vi "灯值调整对话框.vi"() -> ()   [LabVIEW 2016, in "斯坦道氨氮.lvlib"]
uses:
  <vilib>/Plasmionique/MB Master/MB_Master/MB_Master.lvclass
panel:
  out "工作状态:":string
  in  "纯水填充":bool
  out "660 阻值":u16 caption="660 阻值："
  out "520 阻值":u16 caption="520 阻值："
  out "365 阻值":u16 caption="365 阻值："
  in  "停止":bool
  in  "校准":bool
  out "校准状态":u16(ring) caption="调灯状态：" items=["空闲", "校准中"]
  out "当前阻值":u16 caption="当前阻值："
  out "当前光强":u16 caption="当前光强："
  in  "目标光强":u16=3300 caption="目标光强："
  in  "灯类型":enum32{"365", "520", "660"}(radio)=enum."660" caption="灯类型："
  # "365：营养盐\n520：营养盐、氨氮总磷-氨氮光源\n660：总磷、氨氮"
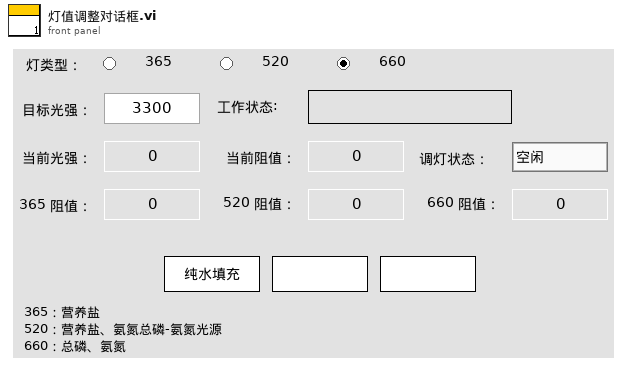
[diagram p1: front panel]
types:
  T1 = cluster{"360 阻值":u16, "520 阻值":u16, "660 阻值":u16}
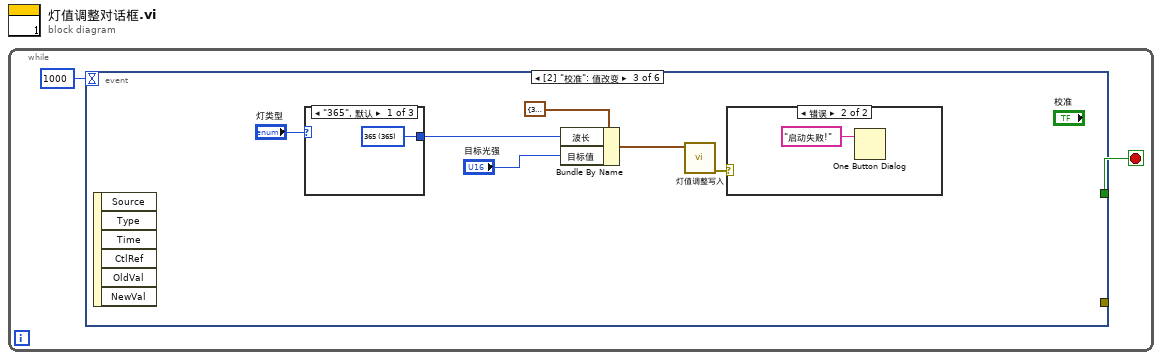
[diagram p0: block diagram]
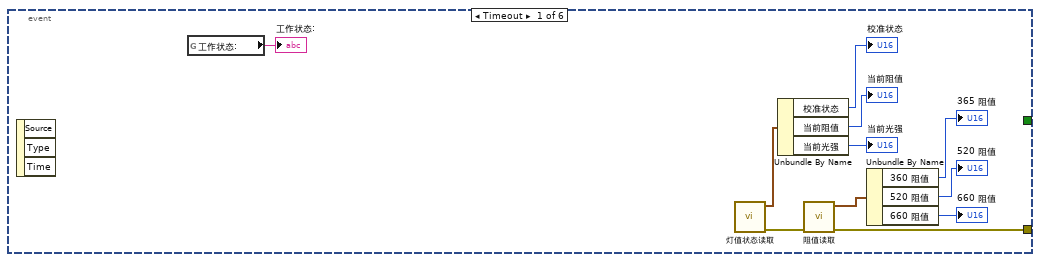
[diagram p2: hidden frame]
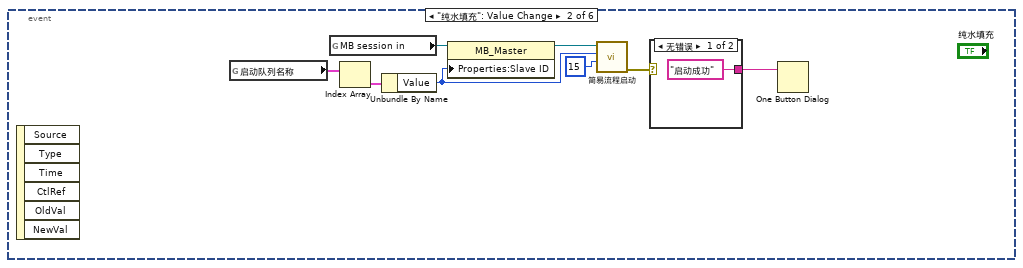
[diagram p3: hidden frame]
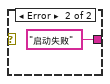
[diagram p4: hidden frame]
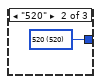
[diagram p6: hidden frame]
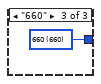
[diagram p7: hidden frame]
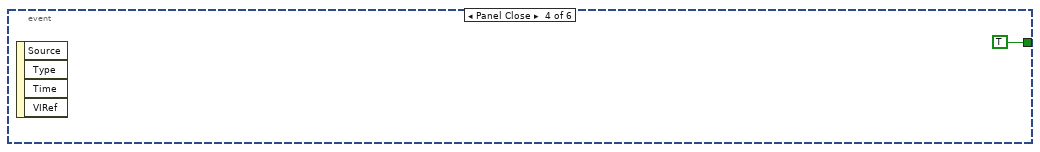
[diagram p8: hidden frame]
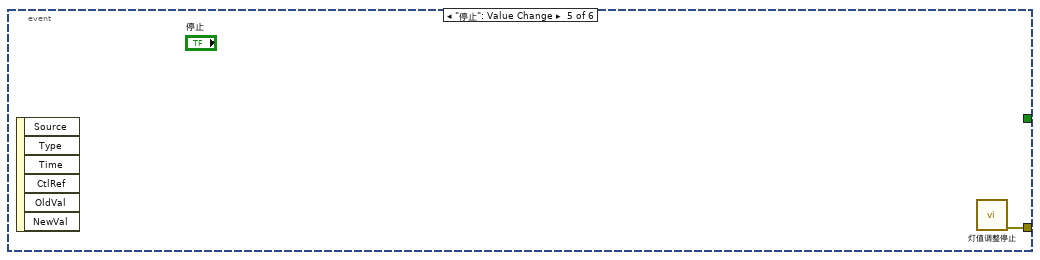
[diagram p9: hidden frame]
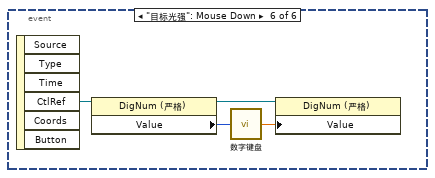
[diagram p10: hidden frame]
diagram:
  n1 = while {
    stop <- w2 stop-if-true
    n2 = event shown="[2] \"校准\": 值改变" {
      selector: _ -> [_ _ _ _ _ _]
      dyn-events: _ -> [_ _ _ _ _ _]
      timeout: 1000 -> [_ _ _ _ _ _]
      tunnel: [_ _ _ TRUE _ _] -> w2
      tunnel: [w4 _ _ _ w35 _] -> _
      event Timeout {
        n3 = event-data() -> ()  [unwired: 1 in, 3 out]
        n4 = global read "VAR总磷总氮全局变量.vi" "工作状态:"() -> (→"工作状态:":string)
        n5 = call "灯值状态读取.vi"() -> ("error out"=w13:errorcluster, "状态值"=w12:cluster{"校准状态":u16, "当前阻值":u16, "当前光强":u16})  [unwired: 10 in]
        n6 = Unbundle By Name(w12) -> ("校准状态"=→"校准状态":u16, "当前阻值"=→"当前阻值":u16, "当前光强"=→"当前光强":u16)
        n7 = call "阻值读取.vi"("error in (no error)"=w13) -> ("error out"=w4:errorcluster, "状态值"=w8:T1)  [unwired: 9 in]
        n8 = Unbundle By Name(w8) -> ("360 阻值"=→"365 阻值":u16, "520 阻值"=→"520 阻值":u16, "660 阻值"=→"660 阻值":u16)
      }
      event "纯水填充": Value Change {
        n9 = event-data() -> ()  [unwired: 1 in, 6 out]
        n10 = global read "总磷总氮断电保存全局变量.vi" "启动队列名称"() -> (w16:cluster{"String":string, "Value":u16}[])
        n11 = global read "VAR总磷总氮全局变量.vi" "MB session in"() -> (w19:refnum<class "MB_Master.lvclass">)
        n12 = Index Array(array=w16) -> (element=w15:cluster{"String":string, "Value":u16})  [unwired: 1 in]
        n13 = Unbundle By Name(w15) -> ("Value"=w14:u16)
        n14 = property class="MB_Master"(reference=w19, "Properties:Slave ID"=w14) -> (reference out=w18:refnum<class "MB_Master.lvclass">)  [unwired: 1 in, 1 out]
        n15 = call "简易流程启动.vi"("简易流程"=15, "参数Id"=w14, "MB session in"=w18) -> ("error out"=w21:errorcluster)  [unwired: 7 in, 1 out]
        n16 = case shown="无错误" w21 {
          tunnel: ["启动成功" "启动失败"] -> w20
          frame No Error {
          }
          frame Error {
          }
        }
        n17 = One Button Dialog(message=w20) -> ()  [unwired: 1 in, 1 out]
      }
      event "校准": Value Change {
        n18 = event-data() -> ()  [unwired: 1 in, 6 out]
        n19 = case shown="\"365\", 默认" "灯类型" {
          tunnel: [w31 w32 w33] -> w24
          frame "365", Default {
            w31 = u16 365 items=["365"=365, "520"=520, "660"=660] ("波长")
          }
          frame "520" {
            w32 = u16 520 items=["365"=365, "520"=520, "660"=660] ("波长")
          }
          frame "660" {
            w33 = u16 660 items=["365"=365, "520"=520, "660"=660] ("波长")
          }
        }
        n20 = Bundle By Name(cluster=cluster{"波长":u16, "ADC":u16, "目标值":u16} {"波长"=365, "ADC"=0, "目标值"=0} ("写入值"), "波长"=w24, "目标值"="目标光强") -> (w26:cluster{"波长":u16, "ADC":u16, "目标值":u16})
        n21 = call "灯值调整写入.vi"("写入值"=w26) -> ("error out"=w27:errorcluster)  [unwired: 10 in]
        n22 = case shown="错误" w27 {
          frame No Error {
          }
          frame Error {
            n23 = One Button Dialog(message="启动失败!" ("消息")) -> ()  [unwired: 1 in, 1 out]
          }
        }
      }
      event Panel Close {
        n24 = event-data() -> ()  [unwired: 1 in, 4 out]
      }
      event "停止": Value Change {
        n25 = event-data() -> ()  [unwired: 1 in, 6 out]
        n26 = call "灯值调整停止.vi"() -> ("error out"=w35:errorcluster)  [unwired: 11 in]
      }
      event "目标光强": Mouse Down {
        n27 = event-data() -> ("CtlRef"=w39:refnum<vi>)  [unwired: 1 in, 5 out]
        n28 = property class="DigNum (严格)"(reference=w39) -> (reference out=w36:refnum<vi>, "Value"=w38:u16)  [unwired: 1 in, 1 out]
        n29 = call "数字键盘.vi"("OldNumber"=w38) -> ("NewNumber"=w37:dbl)
        n30 = property class="DigNum (严格)"(reference=w36, "Value"=w37) -> ()  [unwired: 1 in, 2 out]
      }
    }
  }
